vi "addition.vi"() -> ()   [LabVIEW 2021]
panel:
  out "SUM":dbl
  in  "B":dbl
  in  "A":dbl
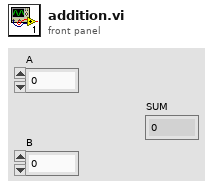
[diagram p1: front panel]
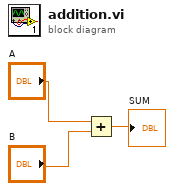
[diagram p0: block diagram]
diagram:
  n1 = Add(x="A", y="B") -> (x+y=→"SUM":dbl)
